vi "RTS Door Ops Sequence Delay.vi"(5 "Door Output Relays":T1, 7 "Station #":u8=1 min=1 max=8 step=1, 8 "error in (no error)":errorcluster, 10 "All Door Opener Ctrl in":T2={"Station 1"={"Station Freezer"={"Time Count (s)"=0.0, "Status"="", "Door State"=FALSE, "Delay"=FALSE, "Chamber 1-1"=[], "Index"=0, "Delay Status"=""}, "Station Cab"={"Time Count (s)"=0.0, "Status"="", "Door State"=FALSE, "Delay"=FALSE, "Chamber 1-1"=[], "Index"=0, "Delay Status"=""}, "Station Slide"={"Time Count (s)"=0.0, "Status"="", "Door State"=FALSE, "Delay"=FALSE, "Chamber 1-1"=[], "Index"=0, "Delay Status"=""}, "1st Complete"=FALSE, "2nd Complete"=FALSE, "3rd Complete"=FALSE}, "Station 2"={"Station Freezer"={"Time Count (s)"=0.0, "Status"="", "Door State"=FALSE, "Delay"=FALSE, "Chamber 1-1"=[], "Index"=0, "Delay Status"=""}, "Station Cab"={"Time Count (s)"=0.0, "Status"="", "Door State"=FALSE, "Delay"=FALSE, "Chamber 1-1"=[], "Index"=0, "Delay Status"=""}, "Station Slide"={"Time Count (s)"=0.0, "Status"="", "Door State"=FALSE, "Delay"=FALSE, "Chamber 1-1"=[], "Index"=0, "Delay Status"=""}, "1st Complete"=FALSE, "2nd Complete"=FALSE, "3rd Complete"=FALSE}, "Station 3"={"Station Freezer"={"Time Count (s)"=0.0, "Status"="", "Door State"=FALSE, "Delay"=FALSE, "Chamber 1-1"=[], "Index"=0, "Delay Status"=""}, "Station Cab"={"Time Count (s)"=0.0, "Status"="", "Door State"=FALSE, "Delay"=FALSE, "Chamber 1-1"=[], "Index"=0, "Delay Status"=""}, "Station Slide"={"Time Count (s)"=0.0, "Status"="", "Door State"=FALSE, "Delay"=FALSE, "Chamber 1-1"=[], "Index"=0, "Delay Status"=""}, "1st Complete"=FALSE, "2nd Complete"=FALSE, "3rd Complete"=FALSE}, "Station 4"={"Station Freezer"={"Time Count (s)"=0.0, "Status"="", "Door State"=FALSE, "Delay"=FALSE, "Chamber 1-1"=[], "Index"=0, "Delay Status"=""}, "Station Cab"={"Time Count (s)"=0.0, "Status"="", "Door State"=FALSE, "Delay"=FALSE, "Chamber 1-1"=[], "Index"=0, "Delay Status"=""}, "Station Slide"={"Time Count (s)"=0.0, "Status"="", "Door State"=FALSE, "Delay"=FALSE, "Chamber 1-1"=[], "Index"=0, "Delay Status"=""}, "1st Complete"=FALSE, "2nd Complete"=FALSE, "3rd Complete"=FALSE}, "Station 5"={"Station Freezer"={"Time Count (s)"=0.0, "Status"="", "Door State"=FALSE, "Delay"=TRUE, "Chamber 1-1"=[], "Index"=0, "Delay Status"=""}, "Station Cab"={"Time Count (s)"=0.0, "Status"="", "Door State"=FALSE, "Delay"=TRUE, "Chamber 1-1"=[], "Index"=0, "Delay Status"=""}, "Station Slide"={"Time Count (s)"=0.0, "Status"="", "Door State"=FALSE, "Delay"=TRUE, "Chamber 1-1"=[], "Index"=0, "Delay Status"=""}, "1st Complete"=FALSE, "2nd Complete"=FALSE, "3rd Complete"=FALSE}, "Station 6"={"Station Freezer"={"Time Count (s)"=0.0, "Status"="", "Door State"=FALSE, "Delay"=TRUE, "Chamber 1-1"=[], "Index"=0, "Delay Status"=""}, "Station Cab"={"Time Count (s)"=0.0, "Status"="", "Door State"=FALSE, "Delay"=TRUE, "Chamber 1-1"=[], "Index"=0, "Delay Status"=""}, "Station Slide"={"Time Count (s)"=0.0, "Status"="", "Door State"=FALSE, "Delay"=TRUE, "Chamber 1-1"=[], "Index"=0, "Delay Status"=""}, "1st Complete"=FALSE, "2nd Complete"=FALSE, "3rd Complete"=FALSE}, "Station 7"={"Station Freezer"={"Time Count (s)"=0.0, "Status"="", "Door State"=FALSE, "Delay"=TRUE, "Chamber 1-1"=[], "Index"=0, "Delay Status"=""}, "Station Cab"={"Time Count (s)"=0.0, "Status"="", "Door State"=FALSE, "Delay"=TRUE, "Chamber 1-1"=[], "Index"=0, "Delay Status"=""}, "Station Slide"={"Time Count (s)"=0.0, "Status"="", "Door State"=FALSE, "Delay"=TRUE, "Chamber 1-1"=[], "Index"=0, "Delay Status"=""}, "1st Complete"=FALSE, "2nd Complete"=FALSE, "3rd Complete"=FALSE}, "Station 8"={"Station Freezer"={"Time Count (s)"=0.0, "Status"="", "Door State"=FALSE, "Delay"=TRUE, "Chamber 1-1"=[], "Index"=0, "Delay Status"=""}, "Station Cab"={"Time Count (s)"=0.0, "Status"="", "Door State"=FALSE, "Delay"=TRUE, "Chamber 1-1"=[], "Index"=0, "Delay Status"=""}, "Station Slide"={"Time Count (s)"=0.0, "Status"="", "Door State"=FALSE, "Delay"=TRUE, "Chamber 1-1"=[], "Index"=0, "Delay Status"=""}, "1st Complete"=FALSE, "2nd Complete"=FALSE, "3rd Complete"=FALSE}} {"Station 8"."Station Slide"."Chamber 1-1"."Start Time" format="%<%X\n%x>T"; "Station 8"."Station Slide"."Chamber 1-1"."End Time" format="%<%X\n%x>T"; "Station 8"."Station Slide"."Time Count (s)" format="%.2f"; "Station 8"."Station Cab"."Chamber 1-1"."Start Time" format="%<%X\n%x>T"; "Station 8"."Station Cab"."Chamber 1-1"."End Time" format="%<%X\n%x>T"; "Station 8"."Station Cab"."Time Count (s)" format="%.2f"; "Station 8"."Station Freezer"."Chamber 1-1"."Start Time" format="%<%X\n%x>T"; "Station 8"."Station Freezer"."Chamber 1-1"."End Time" format="%<%X\n%x>T"; "Station 8"."Station Freezer"."Time Count (s)" format="%.2f"; "Station 7"."Station Slide"."Chamber 1-1"."Start Time" format="%<%X\n%x>T"; "Station 7"."Station Slide"."Chamber 1-1"."End Time" format="%<%X\n%x>T"; "Station 7"."Station Slide"."Time Count (s)" format="%.2f"; "Station 7"."Station Cab"."Chamber 1-1"."Start Time" format="%<%X\n%x>T"; "Station 7"."Station Cab"."Chamber 1-1"."End Time" format="%<%X\n%x>T"; "Station 7"."Station Cab"."Time Count (s)" format="%.2f"; "Station 7"."Station Freezer"."Chamber 1-1"."Start Time" format="%<%X\n%x>T"; "Station 7"."Station Freezer"."Chamber 1-1"."End Time" format="%<%X\n%x>T"; "Station 7"."Station Freezer"."Time Count (s)" format="%.2f"; "Station 6"."Station Slide"."Chamber 1-1"."Start Time" format="%<%X\n%x>T"; "Station 6"."Station Slide"."Chamber 1-1"."End Time" format="%<%X\n%x>T"; "Station 6"."Station Slide"."Time Count (s)" format="%.2f"; "Station 6"."Station Cab"."Chamber 1-1"."Start Time" format="%<%X\n%x>T"; "Station 6"."Station Cab"."Chamber 1-1"."End Time" format="%<%X\n%x>T"; "Station 6"."Station Cab"."Time Count (s)" format="%.2f"; "Station 6"."Station Freezer"."Chamber 1-1"."Start Time" format="%<%X\n%x>T"; "Station 6"."Station Freezer"."Chamber 1-1"."End Time" format="%<%X\n%x>T"; "Station 6"."Station Freezer"."Time Count (s)" format="%.2f"; "Station 5"."Station Slide"."Chamber 1-1"."Start Time" format="%<%X\n%x>T"; "Station 5"."Station Slide"."Chamber 1-1"."End Time" format="%<%X\n%x>T"; "Station 5"."Station Slide"."Time Count (s)" format="%.2f"; "Station 5"."Station Cab"."Chamber 1-1"."Start Time" format="%<%X\n%x>T"; "Station 5"."Station Cab"."Chamber 1-1"."End Time" format="%<%X\n%x>T"; "Station 5"."Station Cab"."Time Count (s)" format="%.2f"; "Station 5"."Station Freezer"."Chamber 1-1"."Start Time" format="%<%X\n%x>T"; "Station 5"."Station Freezer"."Chamber 1-1"."End Time" format="%<%X\n%x>T"; "Station 5"."Station Freezer"."Time Count (s)" format="%.2f"; "Station 4"."Station Slide"."Chamber 1-1"."Start Time" format="%<%X\n%x>T"; "Station 4"."Station Slide"."Chamber 1-1"."End Time" format="%<%X\n%x>T"; "Station 4"."Station Slide"."Time Count (s)" format="%.2f"; "Station 4"."Station Cab"."Chamber 1-1"."Start Time" format="%<%X\n%x>T"; "Station 4"."Station Cab"."Chamber 1-1"."End Time" format="%<%X\n%x>T"; "Station 4"."Station Cab"."Time Count (s)" format="%.2f"; "Station 4"."Station Freezer"."Chamber 1-1"."Start Time" format="%<%X\n%x>T"; "Station 4"."Station Freezer"."Chamber 1-1"."End Time" format="%<%X\n%x>T"; "Station 4"."Station Freezer"."Time Count (s)" format="%.2f"; "Station 3"."Station Slide"."Chamber 1-1"."Start Time" format="%<%X\n%x>T"; "Station 3"."Station Slide"."Chamber 1-1"."End Time" format="%<%X\n%x>T"; "Station 3"."Station Slide"."Time Count (s)" format="%.2f"; "Station 3"."Station Cab"."Chamber 1-1"."Start Time" format="%<%X\n%x>T"; "Station 3"."Station Cab"."Chamber 1-1"."End Time" format="%<%X\n%x>T"; "Station 3"."Station Cab"."Time Count (s)" format="%.2f"; "Station 3"."Station Freezer"."Chamber 1-1"."Start Time" format="%<%X\n%x>T"; "Station 3"."Station Freezer"."Chamber 1-1"."End Time" format="%<%X\n%x>T"; "Station 3"."Station Freezer"."Time Count (s)" format="%.2f"; "Station 2"."Station Slide"."Chamber 1-1"."Start Time" format="%<%X\n%x>T"; "Station 2"."Station Slide"."Chamber 1-1"."End Time" format="%<%X\n%x>T"; "Station 2"."Station Slide"."Time Count (s)" format="%.2f"; "Station 2"."Station Cab"."Chamber 1-1"."Start Time" format="%<%X\n%x>T"; "Station 2"."Station Cab"."Chamber 1-1"."End Time" format="%<%X\n%x>T"; "Station 2"."Station Cab"."Time Count (s)" format="%.2f"; "Station 2"."Station Freezer"."Chamber 1-1"."Start Time" format="%<%X\n%x>T"; "Station 2"."Station Freezer"."Chamber 1-1"."End Time" format="%<%X\n%x>T"; "Station 2"."Station Freezer"."Time Count (s)" format="%.2f"; "Station 1"."Station Slide"."Chamber 1-1"."Start Time" format="%<%X\n%x>T"; "Station 1"."Station Slide"."Chamber 1-1"."End Time" format="%<%X\n%x>T"; "Station 1"."Station Slide"."Time Count (s)" format="%.2f"; "Station 1"."Station Cab"."Chamber 1-1"."Start Time" format="%<%X\n%x>T"; "Station 1"."Station Cab"."Chamber 1-1"."End Time" format="%<%X\n%x>T"; "Station 1"."Station Cab"."Time Count (s)" format="%.2f"; "Station 1"."Station Freezer"."Chamber 1-1"."Start Time" format="%<%X\n%x>T"; "Station 1"."Station Freezer"."Chamber 1-1"."End Time" format="%<%X\n%x>T"; "Station 1"."Station Freezer"."Time Count (s)" format="%.2f"}, 11 "Wago ModBus Connection":refnum<class "Modbus Master.lvclass">) -> (0 "error out":errorcluster, 2 "All Door Opener Ctrl out":T2={"Station 1"={"Station Freezer"={"Time Count (s)"=0.0, "Status"="", "Door State"=FALSE, "Delay"=FALSE, "Chamber 1-1"=[], "Index"=0, "Delay Status"=""}, "Station Cab"={"Time Count (s)"=0.0, "Status"="", "Door State"=FALSE, "Delay"=FALSE, "Chamber 1-1"=[], "Index"=0, "Delay Status"=""}, "Station Slide"={"Time Count (s)"=0.0, "Status"="", "Door State"=FALSE, "Delay"=FALSE, "Chamber 1-1"=[], "Index"=0, "Delay Status"=""}, "1st Complete"=FALSE, "2nd Complete"=FALSE, "3rd Complete"=FALSE}, "Station 2"={"Station Freezer"={"Time Count (s)"=0.0, "Status"="", "Door State"=FALSE, "Delay"=FALSE, "Chamber 1-1"=[], "Index"=0, "Delay Status"=""}, "Station Cab"={"Time Count (s)"=0.0, "Status"="", "Door State"=FALSE, "Delay"=FALSE, "Chamber 1-1"=[], "Index"=0, "Delay Status"=""}, "Station Slide"={"Time Count (s)"=0.0, "Status"="", "Door State"=FALSE, "Delay"=FALSE, "Chamber 1-1"=[], "Index"=0, "Delay Status"=""}, "1st Complete"=FALSE, "2nd Complete"=FALSE, "3rd Complete"=FALSE}, "Station 3"={"Station Freezer"={"Time Count (s)"=0.0, "Status"="", "Door State"=FALSE, "Delay"=FALSE, "Chamber 1-1"=[], "Index"=0, "Delay Status"=""}, "Station Cab"={"Time Count (s)"=0.0, "Status"="", "Door State"=FALSE, "Delay"=FALSE, "Chamber 1-1"=[], "Index"=0, "Delay Status"=""}, "Station Slide"={"Time Count (s)"=0.0, "Status"="", "Door State"=FALSE, "Delay"=FALSE, "Chamber 1-1"=[], "Index"=0, "Delay Status"=""}, "1st Complete"=FALSE, "2nd Complete"=FALSE, "3rd Complete"=FALSE}, "Station 4"={"Station Freezer"={"Time Count (s)"=0.0, "Status"="", "Door State"=FALSE, "Delay"=FALSE, "Chamber 1-1"=[], "Index"=0, "Delay Status"=""}, "Station Cab"={"Time Count (s)"=0.0, "Status"="", "Door State"=FALSE, "Delay"=FALSE, "Chamber 1-1"=[], "Index"=0, "Delay Status"=""}, "Station Slide"={"Time Count (s)"=0.0, "Status"="", "Door State"=FALSE, "Delay"=FALSE, "Chamber 1-1"=[], "Index"=0, "Delay Status"=""}, "1st Complete"=FALSE, "2nd Complete"=FALSE, "3rd Complete"=FALSE}, "Station 5"={"Station Freezer"={"Time Count (s)"=0.0, "Status"="", "Door State"=FALSE, "Delay"=TRUE, "Chamber 1-1"=[], "Index"=0, "Delay Status"=""}, "Station Cab"={"Time Count (s)"=0.0, "Status"="", "Door State"=FALSE, "Delay"=TRUE, "Chamber 1-1"=[], "Index"=0, "Delay Status"=""}, "Station Slide"={"Time Count (s)"=0.0, "Status"="", "Door State"=FALSE, "Delay"=TRUE, "Chamber 1-1"=[], "Index"=0, "Delay Status"=""}, "1st Complete"=FALSE, "2nd Complete"=FALSE, "3rd Complete"=FALSE}, "Station 6"={"Station Freezer"={"Time Count (s)"=0.0, "Status"="", "Door State"=FALSE, "Delay"=TRUE, "Chamber 1-1"=[], "Index"=0, "Delay Status"=""}, "Station Cab"={"Time Count (s)"=0.0, "Status"="", "Door State"=FALSE, "Delay"=TRUE, "Chamber 1-1"=[], "Index"=0, "Delay Status"=""}, "Station Slide"={"Time Count (s)"=0.0, "Status"="", "Door State"=FALSE, "Delay"=TRUE, "Chamber 1-1"=[], "Index"=0, "Delay Status"=""}, "1st Complete"=FALSE, "2nd Complete"=FALSE, "3rd Complete"=FALSE}, "Station 7"={"Station Freezer"={"Time Count (s)"=0.0, "Status"="", "Door State"=FALSE, "Delay"=TRUE, "Chamber 1-1"=[], "Index"=0, "Delay Status"=""}, "Station Cab"={"Time Count (s)"=0.0, "Status"="", "Door State"=FALSE, "Delay"=TRUE, "Chamber 1-1"=[], "Index"=0, "Delay Status"=""}, "Station Slide"={"Time Count (s)"=0.0, "Status"="", "Door State"=FALSE, "Delay"=TRUE, "Chamber 1-1"=[], "Index"=0, "Delay Status"=""}, "1st Complete"=FALSE, "2nd Complete"=FALSE, "3rd Complete"=FALSE}, "Station 8"={"Station Freezer"={"Time Count (s)"=0.0, "Status"="", "Door State"=FALSE, "Delay"=TRUE, "Chamber 1-1"=[], "Index"=0, "Delay Status"=""}, "Station Cab"={"Time Count (s)"=0.0, "Status"="", "Door State"=FALSE, "Delay"=TRUE, "Chamber 1-1"=[], "Index"=0, "Delay Status"=""}, "Station Slide"={"Time Count (s)"=0.0, "Status"="", "Door State"=FALSE, "Delay"=TRUE, "Chamber 1-1"=[], "Index"=0, "Delay Status"=""}, "1st Complete"=FALSE, "2nd Complete"=FALSE, "3rd Complete"=FALSE}} {"Station 8"."Station Slide"."Chamber 1-1"."Start Time" format="%<%X\n%x>T"; "Station 8"."Station Slide"."Chamber 1-1"."End Time" format="%<%X\n%x>T"; "Station 8"."Station Slide"."Time Count (s)" format="%.2f"; "Station 8"."Station Cab"."Chamber 1-1"."Start Time" format="%<%X\n%x>T"; "Station 8"."Station Cab"."Chamber 1-1"."End Time" format="%<%X\n%x>T"; "Station 8"."Station Cab"."Time Count (s)" format="%.2f"; "Station 8"."Station Freezer"."Chamber 1-1"."Start Time" format="%<%X\n%x>T"; "Station 8"."Station Freezer"."Chamber 1-1"."End Time" format="%<%X\n%x>T"; "Station 8"."Station Freezer"."Time Count (s)" format="%.2f"; "Station 7"."Station Slide"."Chamber 1-1"."Start Time" format="%<%X\n%x>T"; "Station 7"."Station Slide"."Chamber 1-1"."End Time" format="%<%X\n%x>T"; "Station 7"."Station Slide"."Time Count (s)" format="%.2f"; "Station 7"."Station Cab"."Chamber 1-1"."Start Time" format="%<%X\n%x>T"; "Station 7"."Station Cab"."Chamber 1-1"."End Time" format="%<%X\n%x>T"; "Station 7"."Station Cab"."Time Count (s)" format="%.2f"; "Station 7"."Station Freezer"."Chamber 1-1"."Start Time" format="%<%X\n%x>T"; "Station 7"."Station Freezer"."Chamber 1-1"."End Time" format="%<%X\n%x>T"; "Station 7"."Station Freezer"."Time Count (s)" format="%.2f"; "Station 6"."Station Slide"."Chamber 1-1"."Start Time" format="%<%X\n%x>T"; "Station 6"."Station Slide"."Chamber 1-1"."End Time" format="%<%X\n%x>T"; "Station 6"."Station Slide"."Time Count (s)" format="%.2f"; "Station 6"."Station Cab"."Chamber 1-1"."Start Time" format="%<%X\n%x>T"; "Station 6"."Station Cab"."Chamber 1-1"."End Time" format="%<%X\n%x>T"; "Station 6"."Station Cab"."Time Count (s)" format="%.2f"; "Station 6"."Station Freezer"."Chamber 1-1"."Start Time" format="%<%X\n%x>T"; "Station 6"."Station Freezer"."Chamber 1-1"."End Time" format="%<%X\n%x>T"; "Station 6"."Station Freezer"."Time Count (s)" format="%.2f"; "Station 5"."Station Slide"."Chamber 1-1"."Start Time" format="%<%X\n%x>T"; "Station 5"."Station Slide"."Chamber 1-1"."End Time" format="%<%X\n%x>T"; "Station 5"."Station Slide"."Time Count (s)" format="%.2f"; "Station 5"."Station Cab"."Chamber 1-1"."Start Time" format="%<%X\n%x>T"; "Station 5"."Station Cab"."Chamber 1-1"."End Time" format="%<%X\n%x>T"; "Station 5"."Station Cab"."Time Count (s)" format="%.2f"; "Station 5"."Station Freezer"."Chamber 1-1"."Start Time" format="%<%X\n%x>T"; "Station 5"."Station Freezer"."Chamber 1-1"."End Time" format="%<%X\n%x>T"; "Station 5"."Station Freezer"."Time Count (s)" format="%.2f"; "Station 4"."Station Slide"."Chamber 1-1"."Start Time" format="%<%X\n%x>T"; "Station 4"."Station Slide"."Chamber 1-1"."End Time" format="%<%X\n%x>T"; "Station 4"."Station Slide"."Time Count (s)" format="%.2f"; "Station 4"."Station Cab"."Chamber 1-1"."Start Time" format="%<%X\n%x>T"; "Station 4"."Station Cab"."Chamber 1-1"."End Time" format="%<%X\n%x>T"; "Station 4"."Station Cab"."Time Count (s)" format="%.2f"; "Station 4"."Station Freezer"."Chamber 1-1"."Start Time" format="%<%X\n%x>T"; "Station 4"."Station Freezer"."Chamber 1-1"."End Time" format="%<%X\n%x>T"; "Station 4"."Station Freezer"."Time Count (s)" format="%.2f"; "Station 3"."Station Slide"."Chamber 1-1"."Start Time" format="%<%X\n%x>T"; "Station 3"."Station Slide"."Chamber 1-1"."End Time" format="%<%X\n%x>T"; "Station 3"."Station Slide"."Time Count (s)" format="%.2f"; "Station 3"."Station Cab"."Chamber 1-1"."Start Time" format="%<%X\n%x>T"; "Station 3"."Station Cab"."Chamber 1-1"."End Time" format="%<%X\n%x>T"; "Station 3"."Station Cab"."Time Count (s)" format="%.2f"; "Station 3"."Station Freezer"."Chamber 1-1"."Start Time" format="%<%X\n%x>T"; "Station 3"."Station Freezer"."Chamber 1-1"."End Time" format="%<%X\n%x>T"; "Station 3"."Station Freezer"."Time Count (s)" format="%.2f"; "Station 2"."Station Slide"."Chamber 1-1"."Start Time" format="%<%X\n%x>T"; "Station 2"."Station Slide"."Chamber 1-1"."End Time" format="%<%X\n%x>T"; "Station 2"."Station Slide"."Time Count (s)" format="%.2f"; "Station 2"."Station Cab"."Chamber 1-1"."Start Time" format="%<%X\n%x>T"; "Station 2"."Station Cab"."Chamber 1-1"."End Time" format="%<%X\n%x>T"; "Station 2"."Station Cab"."Time Count (s)" format="%.2f"; "Station 2"."Station Freezer"."Chamber 1-1"."Start Time" format="%<%X\n%x>T"; "Station 2"."Station Freezer"."Chamber 1-1"."End Time" format="%<%X\n%x>T"; "Station 2"."Station Freezer"."Time Count (s)" format="%.2f"; "Station 1"."Station Slide"."Chamber 1-1"."Start Time" format="%<%X\n%x>T"; "Station 1"."Station Slide"."Chamber 1-1"."End Time" format="%<%X\n%x>T"; "Station 1"."Station Slide"."Time Count (s)" format="%.2f"; "Station 1"."Station Cab"."Chamber 1-1"."Start Time" format="%<%X\n%x>T"; "Station 1"."Station Cab"."Chamber 1-1"."End Time" format="%<%X\n%x>T"; "Station 1"."Station Cab"."Time Count (s)" format="%.2f"; "Station 1"."Station Freezer"."Chamber 1-1"."Start Time" format="%<%X\n%x>T"; "Station 1"."Station Freezer"."Chamber 1-1"."End Time" format="%<%X\n%x>T"; "Station 1"."Station Freezer"."Time Count (s)" format="%.2f"}, 3 "Modbus Master Out":refnum<class "Modbus Master.lvclass">)   [LabVIEW 2016]
uses:
  Type Definitions/RTS All Station Door Opener Ctrl.ctl
  Type Definitions/RTS Station Relay Ops.ctl
  Type Definitions/RTS Door Opener Indicator.ctl
  Type Definitions/RTS Door Ops Client.ctl
  Type Definitions/RTS Door Opening Schedule.ctl
  Type Definitions/RTS Door Ops Sequence.ctl
  Drivers/WAGO 750-881/Type Definitions/Wago Door Relays.ctl
  <vilib>/NI/Modbus Library/API/Master/Modbus Master.lvclass
panel:
  # "Chamber Conditions:"
  # "Chamber Conditions:"
  # "Chamber Conditions:"
  # "Chamber Conditions:"
  # "Chamber Conditions:"
  # "Chamber Conditions:"
  # "Chamber Conditions:"
  # "Chamber Conditions:"
  # "Chamber Conditions:"
  # "Chamber Conditions:"
  # "Chamber Conditions:"
  # "Chamber Conditions:"
  # "Chamber Conditions:"
  # "Chamber Conditions:"
  # "Chamber Conditions:"
  # "Chamber Conditions:"
  # "Chamber Conditions:"
  # "Chamber Conditions:"
  # "Chamber Conditions:"
  # "Chamber Conditions:"
  # "Chamber Conditions:"
  # "Chamber Conditions:"
  # "Chamber Conditions:"
  # "Chamber Conditions:"
  # "Chamber Conditions:"
  # "Chamber Conditions:"
  # "Chamber Conditions:"
  # "Chamber Conditions:"
  # "Chamber Conditions:"
  # "Chamber Conditions:"
  # "Chamber Conditions:"
  # "Chamber Conditions:"
  # "Chamber Conditions:"
  # "Chamber Conditions:"
  # "Chamber Conditions:"
  # "Chamber Conditions:"
  # "Chamber Conditions:"
  # "Chamber Conditions:"
  # "Chamber Conditions:"
  # "Chamber Conditions:"
  # "Chamber Conditions:"
  # "Chamber Conditions:"
  # "Chamber Conditions:"
  # "Chamber Conditions:"
  # "Chamber Conditions:"
  # "Chamber Conditions:"
  # "Chamber Conditions:"
  # "Chamber Conditions:"
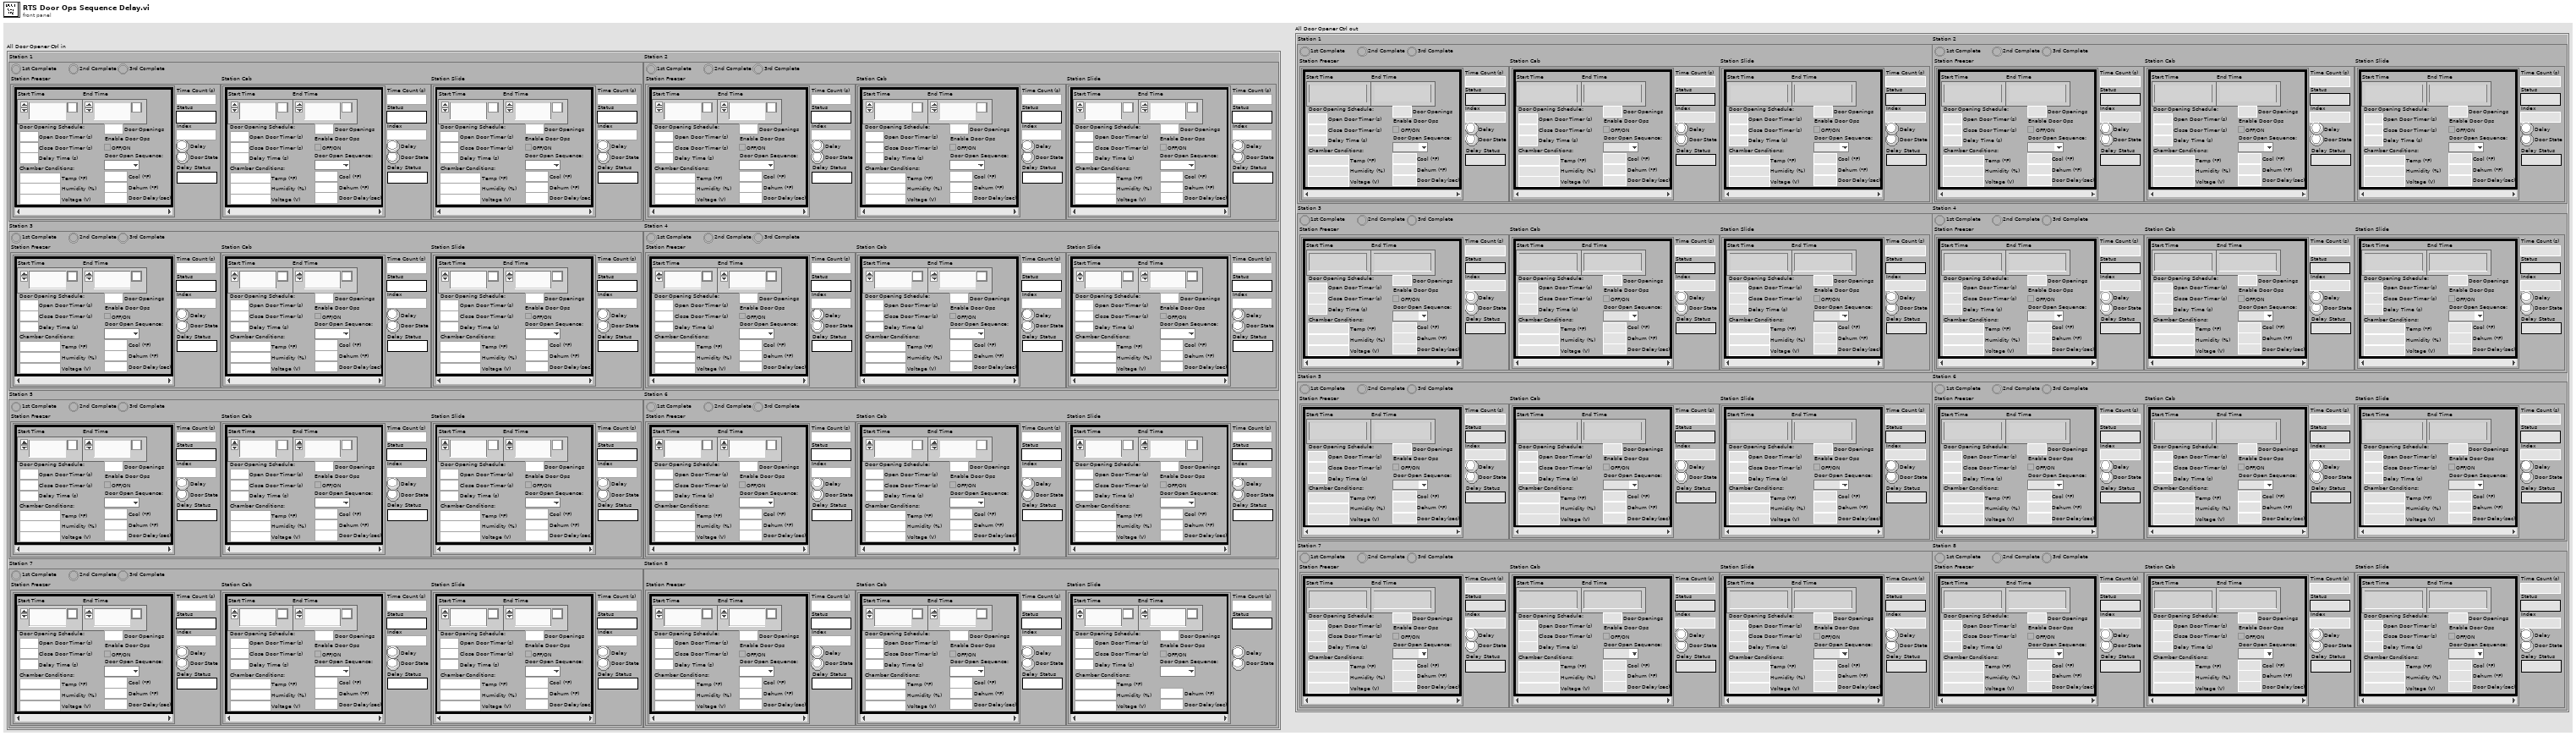
[diagram p1: front panel]
types:
  T1 = typedef "Wago Door Relays.ctl" = cluster{"Station 1 Freezer":bool, "Station 1 Cab":bool, "Station 1 Slide":bool, "Station 2 Freezer":bool, "Station 2 Cab":bool, "Station 2 Slide":bool, "Station 3 Freezer":bool, "Station 3 Cab":bool, "Station 3 Slide":bool, "Station 4 Freezer":bool, "Station 4 Cab":bool, "Station 4 Slide":bool, "Station 5 Freezer":bool, "Station 5 Cab":bool, "Station 5 Slide":bool, "Station 6 Freezer":bool, "Station 6 Cab":bool, "Station 6 Slide":bool, "Station 7 Freezer":bool, "Station 7 Cab":bool, "Station 7 Slide":bool, "Station 8 Freezer":bool, "Station 8 Cab":bool, "Station 8 Slide":bool, "Door Opener Enable":bool}
  T2 = typedef "RTS All Station Door Opener Ctrl.ctl" = cluster{"Station 1":T3, "Station 2":T3, "Station 3":T3, "Station 4":T3, "Station 5":T3, "Station 6":T3, "Station 7":T3, "Station 8":T3}
  T3 = typedef "RTS Station Relay Ops.ctl" = cluster{"Station Freezer":T4, "Station Cab":T4, "Station Slide":T4, "1st Complete":bool, "2nd Complete":bool, "3rd Complete":bool}
  T4 = typedef "RTS Door Opener Indicator.ctl" = cluster{"Time Count (s)":dbl, "Status":string, "Door State":bool, "Delay":bool, "Chamber 1-1":T5[], "Index":i32, "Delay Status":string}
  T5 = typedef "RTS Door Ops Client.ctl" = cluster{"End Time":timestamp, "Start Time":timestamp, "Door Opening Schedule:":T6, "Enable Door Ops":bool, "Door Openings":u32, "Temp (°F)":dbl, "Humidity (%)":dbl, "Voltage (V)":dbl, "Door Open Sequence:":T7, "Door Delay(sec)":dbl, "Dehum (°F)":dbl, "Cool (°F)":dbl}
  T6 = typedef "RTS Door Opening Schedule.ctl" = cluster{"Open Door Timer (s)":dbl, "Delay Time (s)":dbl, "Close Door Timer (s)":dbl}
  T7 = typedef "RTS Door Ops Sequence.ctl" = enum16{"", "1st", "2nd", "3rd"}
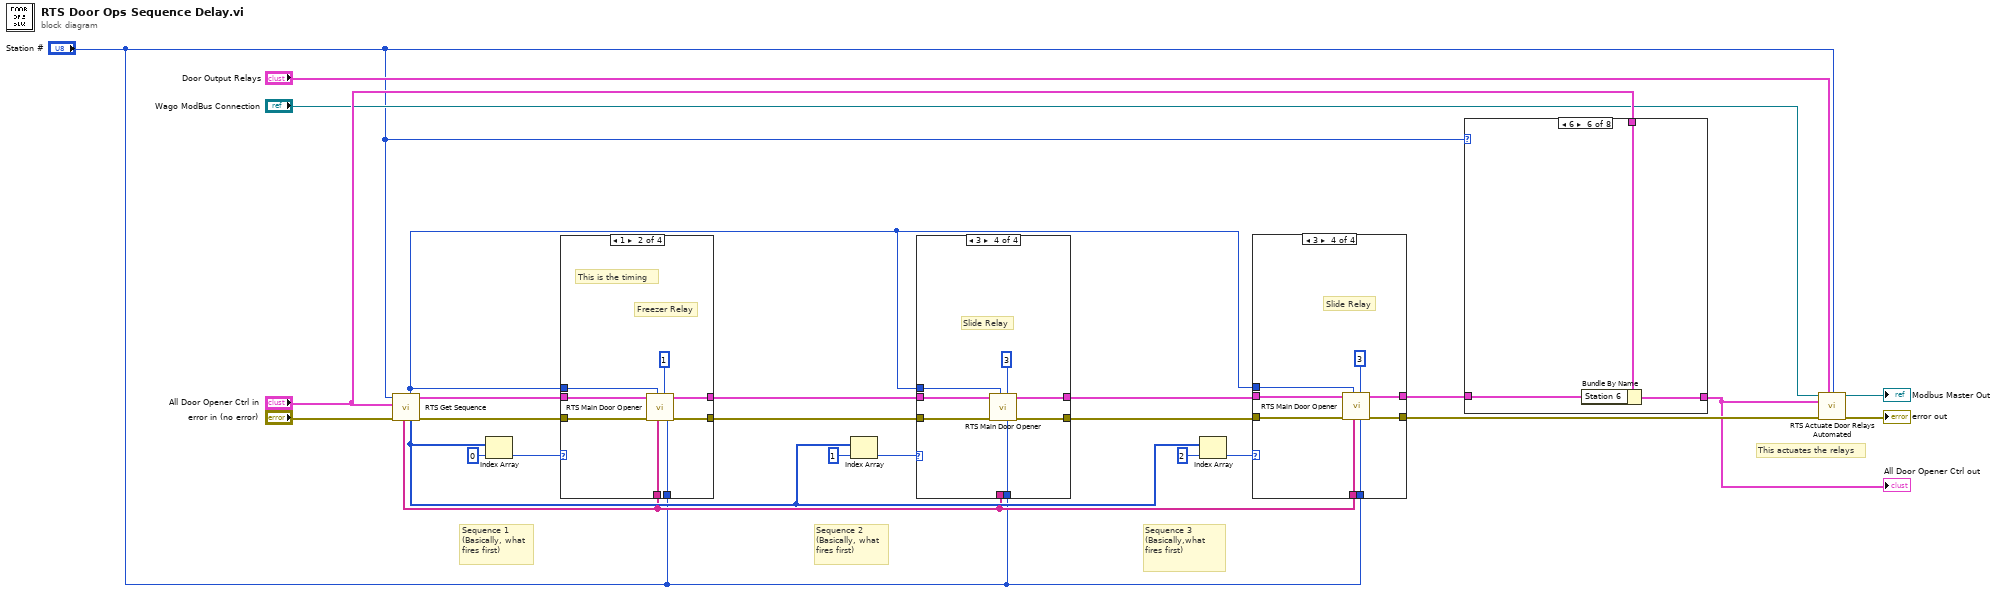
[diagram p0: block diagram]
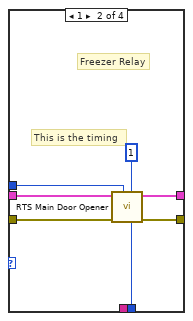
[diagram p3: hidden frame]
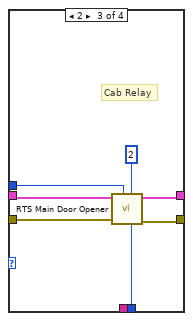
[diagram p4: hidden frame]
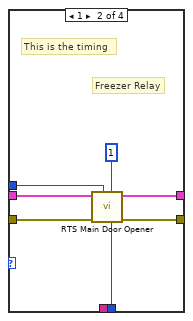
[diagram p6: hidden frame]
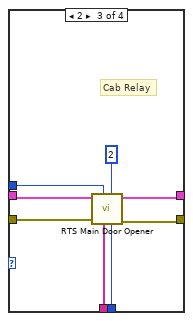
[diagram p7: hidden frame]
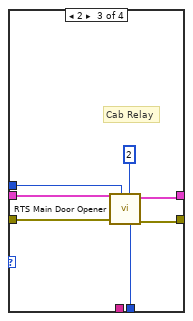
[diagram p9: hidden frame]
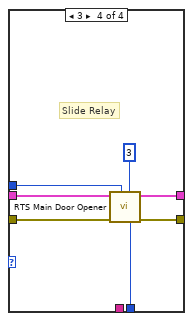
[diagram p10: hidden frame]
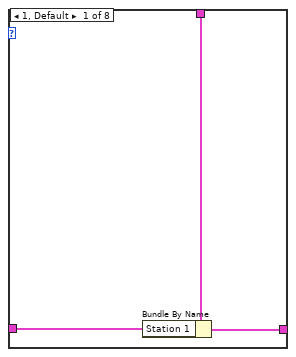
[diagram p11: hidden frame]
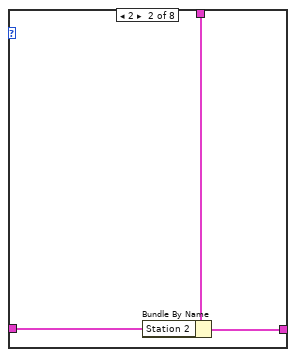
[diagram p12: hidden frame]
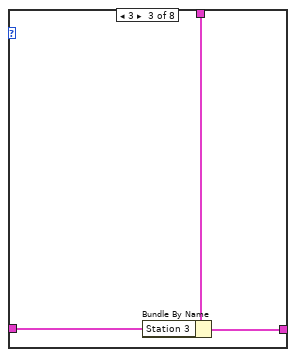
[diagram p13: hidden frame]
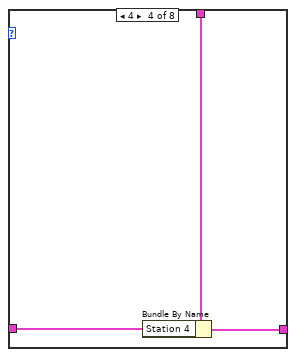
[diagram p14: hidden frame]
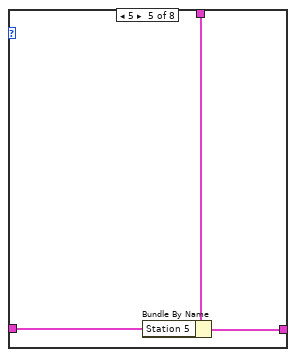
[diagram p15: hidden frame]
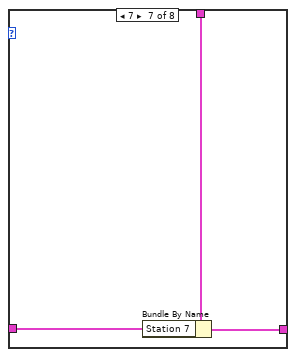
[diagram p16: hidden frame]
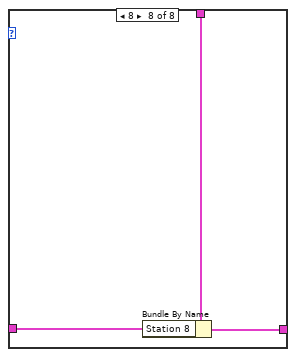
[diagram p17: hidden frame]
diagram:
  # "Sequence 3 (Basically,what fires first)"
  # "Sequence 2\n(Basically, what\nfires first)"
  # "Sequence 1 \n(Basically, what\nfires first)"
  # "This actuates the relays"
  n1 = call "RTS Get Sequence.vi"("Error In"="error in (no error)", "All Door Opener Ctrl in"="All Door Opener Ctrl in", "Station #"="Station #") -> ("Error Out"=w19:errorcluster, "Station 1-8 Data"=w12:T3, "Run Order"=w10:u8[], "Array Size"=w2:i32, "Current Status"=w3:string[])  [unwired: 4 in]
  n2 = Index Array(array=w10, index=0) -> (element=w17:u8)
  n3 = case shown="1" w17 {
    tunnel: w2 -> [_ w35 w39 w45]
    tunnel: [w27 w34 w37 w44] -> w7
    tunnel: w12 -> [w27 w32 w38 w46]
    tunnel: w19 -> [w26 w31 w41 w47]
    tunnel: [w26 w30 w40 w48] -> w14
    tunnel: w3 -> [_ w29 _ _]
    tunnel: "Station #" -> [_ w28 w36 w43]
    frame Default {
    }
    frame 1 {
      # "Freezer Relay"
      # "This is the timing"
      n4 = call "RTS Main Door Opener.vi"("Station #"=w28, "Relay Number"=u8 1, "Current Status"=w29, "Array Size"=w35, "Error In"=w31, "Station 1-8 Data"=w32) -> ("Error Out"=w30:errorcluster, "Station Cluster"=w34:T3)  [unwired: 4 in]
    }
    frame 2 {
      # "Cab Relay"
      n5 = call "RTS Main Door Opener.vi"("Station #"=w36, "Relay Number"=u8 2, "Array Size"=w39, "Error In"=w41, "Station 1-8 Data"=w38) -> ("Error Out"=w40:errorcluster, "Station Cluster"=w37:T3)  [unwired: 5 in]
    }
    frame 3 {
      # "Slide Relay"
      n6 = call "RTS Main Door Opener.vi"("Station #"=w43, "Relay Number"=u8 3, "Array Size"=w45, "Error In"=w47, "Station 1-8 Data"=w46) -> ("Error Out"=w48:errorcluster, "Station Cluster"=w44:T3)  [unwired: 5 in]
    }
  }
  n7 = Index Array(array=w10, index=1) -> (element=w15:u8)
  n8 = case shown="3" w15 {
    tunnel: w2 -> [_ w58 w62 w69]
    tunnel: [w50 w57 w61 w68] -> w6
    tunnel: w7 -> [w50 w55 w63 w70]
    tunnel: w14 -> [w51 w54 w65 w71]
    tunnel: [w51 w53 w64 w72] -> w13
    tunnel: w3 -> [_ _ w60 _]
    tunnel: "Station #" -> [_ w52 w59 w67]
    frame Default {
    }
    frame 1 {
      # "Freezer Relay"
      # "This is the timing"
      n9 = call "RTS Main Door Opener.vi"("Station #"=w52, "Relay Number"=u8 1, "Array Size"=w58, "Error In"=w54, "Station 1-8 Data"=w55) -> ("Error Out"=w53:errorcluster, "Station Cluster"=w57:T3)  [unwired: 5 in]
    }
    frame 2 {
      # "Cab Relay"
      n10 = call "RTS Main Door Opener.vi"("Station #"=w59, "Relay Number"=u8 2, "Current Status"=w60, "Array Size"=w62, "Error In"=w65, "Station 1-8 Data"=w63) -> ("Error Out"=w64:errorcluster, "Station Cluster"=w61:T3)  [unwired: 4 in]
    }
    frame 3 {
      # "Slide Relay"
      n11 = call "RTS Main Door Opener.vi"("Station #"=w67, "Relay Number"=u8 3, "Array Size"=w69, "Error In"=w71, "Station 1-8 Data"=w70) -> ("Error Out"=w72:errorcluster, "Station Cluster"=w68:T3)  [unwired: 5 in]
    }
  }
  n12 = Index Array(array=w10, index=2) -> (element=w9:u8)
  n13 = case shown="3" w9 {
    tunnel: w2 -> [_ w82 w85 w93]
    tunnel: [w74 w81 w84 w92] -> w5
    tunnel: w6 -> [w74 w79 w86 w94]
    tunnel: w13 -> [w75 w78 w88 w95]
    tunnel: [w75 w77 w87 w96] -> w8
    tunnel: w3 -> [_ _ _ w91]
    tunnel: "Station #" -> [_ w76 w83 w90]
    frame Default {
    }
    frame 1 {
      # "Freezer Relay"
      # "This is the timing"
      n14 = call "RTS Main Door Opener.vi"("Station #"=w76, "Relay Number"=u8 1, "Array Size"=w82, "Error In"=w78, "Station 1-8 Data"=w79) -> ("Error Out"=w77:errorcluster, "Station Cluster"=w81:T3)  [unwired: 5 in]
    }
    frame 2 {
      # "Cab Relay"
      n15 = call "RTS Main Door Opener.vi"("Station #"=w83, "Relay Number"=u8 2, "Array Size"=w85, "Error In"=w88, "Station 1-8 Data"=w86) -> ("Error Out"=w87:errorcluster, "Station Cluster"=w84:T3)  [unwired: 5 in]
    }
    frame 3 {
      # "Slide Relay"
      n16 = call "RTS Main Door Opener.vi"("Station #"=w90, "Relay Number"=u8 3, "Current Status"=w91, "Array Size"=w93, "Error In"=w95, "Station 1-8 Data"=w94) -> ("Error Out"=w96:errorcluster, "Station Cluster"=w92:T3)  [unwired: 4 in]
    }
  }
  n17 = case shown="6" "Station #" {
    tunnel: [w100 w102 w105 w108 w111 w114 w117 w120] -> w4
    tunnel: "All Door Opener Ctrl in" -> [w99 w103 w106 w109 w112 w115 w118 w121]
    tunnel: w5 -> [w98 w101 w104 w107 w110 w113 w116 w119]
    frame 1, Default {
      n18 = Bundle By Name(cluster=w99, "Station 1"=w98) -> (w100:T2)
    }
    frame 2 {
      n19 = Bundle By Name(cluster=w103, "Station 2"=w101) -> (w102:T2)
    }
    frame 3 {
      n20 = Bundle By Name(cluster=w106, "Station 3"=w104) -> (w105:T2)
    }
    frame 4 {
      n21 = Bundle By Name(cluster=w109, "Station 4"=w107) -> (w108:T2)
    }
    frame 5 {
      n22 = Bundle By Name(cluster=w112, "Station 5"=w110) -> (w111:T2)
    }
    frame 6 {
      n23 = Bundle By Name(cluster=w115, "Station 6"=w113) -> (w114:T2)
    }
    frame 7 {
      n24 = Bundle By Name(cluster=w118, "Station 7"=w116) -> (w117:T2)
    }
    frame 8 {
      n25 = Bundle By Name(cluster=w121, "Station 8"=w119) -> (w120:T2)
    }
  }
  "All Door Opener Ctrl out" <- w4
  n26 = call "RTS Actuate Door Relays Automated.vi"("Wago ModBus Connection"="Wago ModBus Connection", "Door Output Relays"="Door Output Relays", "Station #"="Station #", "All Door Opener Ctrl out"=w4, "Error In"=w8) -> ("Modbus Master Out"=→"Modbus Master Out":refnum<class "Modbus Master.lvclass">, "Error Out"=→"error out":errorcluster)  [unwired: 9 in]
